vi "WS_RS485ETH_open.vi"(8 "error in":errorcluster, 10 "port":u16=4196, 11 "ip_addr":string="192.168.24.133") -> (0 "error out":errorcluster, 3 "conn_id":refnum<k5>, 4 "status":bool)   [LabVIEW 2019]
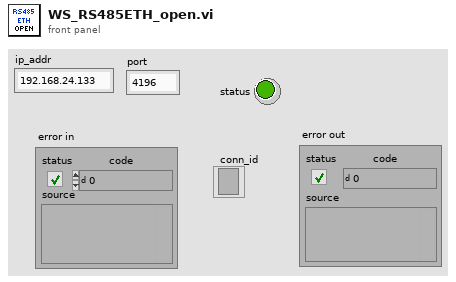
[diagram p1: front panel]
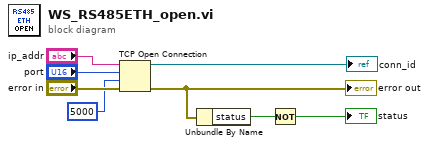
[diagram p0: block diagram]
diagram:
  n1 = TCP Open Connection(address="ip_addr", remote port or service name="port", timeout ms (60000)=5000, error in (no error)="error in") -> (connection ID=→"conn_id":refnum<k5>, error out=w4:errorcluster)  [unwired: 1 in]
  "error out" <- w4
  n2 = Unbundle By Name(w4) -> ("status"=w3:bool)
  n3 = Not(x=w3) -> (.not. x?=→"status":bool)
